vi "Begin.vi"   [LabVIEW 2020]
doc: "Called before other user functions, this VI is expected to open initial I/O refnums, load in file data, and do all program initialization. Notice that the <B>error out</B> terminal is simply used for data flow. Wiring it to other structures or subVIs ensures that this VI runs first."
uses:
  <vilib>/Rock Robotics/WPI/DriverStation/WPI_DriverStationRobotMode2.ctl
  <vilib>/Rock Robotics/WPI/Joystick/WPI_JoystickDeviceEnum.ctl
  <vilib>/Rock Robotics/WPI/ThirdParty/REV Robotics/REVLib/Typedef/Spark MAX Control Type.ctl
  Robot Global Data.vi
  <vilib>/Rock Robotics/WPI/ThirdParty/Phoenix-LabVIEW/CANCoder/Get/CTRE_Phoenix_CANcoder_GetSensorData.vi
  <vilib>/Rock Robotics/WPI/ThirdParty/Phoenix-LabVIEW/CANCoder/Set/CTRE_Phoenix_CANcoder_SetPosition.vi
types:
  T1 = typedef "Spark MAX Control Type.ctl" = enum16{"Percent VBus", "Voltage", "Velocity", "Position", "Smart Motion", "Current", "Smart Velocity"}
  T2 = typedef "WPI_JoystickDeviceEnum.ctl" = enum16{"USB 0", "USB 1", "USB 2", "USB 3", "USB 4", "USB 5"}
  T3 = typedef "WPI_DriverStationRobotMode2.ctl" = enum16{"Autonomous Disabled", "Autonomous Enabled", "Teleop Disabled", "Teleop Enabled", "Disconnected", "Finish", "Test Disabled", "Test Enabled", "Emergency Stopped"}
  T4 = typedef "WPI_MotorControlDeviceRef.ctl" = cluster{"DeviceStatus":errorcluster, "Type":T5, "PWM":cluster{"PWM Channel":T6, "DeadBand":T7}, "CAN":cluster{"Device Number":u8, "SetOutput VI Ref":variant, "GetOutput VI Ref":variant, "Enable VI Ref":variant, "Disable VI Ref":variant, "Data":variant}, "Invert":bool, "DIO PWM":cluster{"PWM \"Enable\" Channel":T6, "DIOChannel":T8, "PWM Rate":dbl}}
  T5 = typedef "WPI_MotorControlType.ctl" = enum16{"PWM", "CAN", "DIO PWM"}
  T6 = typedef "FPGA_DIOPWMChannel.ctl" = enum8{"PWM 0", "PWM 1", "PWM 2", "PWM 3", "PWM 4", "PWM 5", "PWM 6", "PWM 7", "PWM 8", "PWM 9", "PWM MXP 0", "PWM MXP 1", "PWM MXP 2", "PWM MXP 3", "PWM MXP 4", "PWM MXP 5", "PWM MXP 6", "PWM MXP 7", "PWM MXP 8", "PWM MXP 9", "Invalid"}
  T7 = typedef "WPI_PWMDeadband.ctl" = cluster{"Name":string, "maxPositivePwm":i32, "minPositivePwm":i32, "centerPwm":i32, "maxNegativePwm":i32, "minNegativePwm":i32, "angularRange":u16}
  T8 = typedef "FPGA_DIOChannel.ctl" = enum8{"DIO 0", "DIO 1", "DIO 2", "DIO 3", "DIO 4", "DIO 5", "DIO 6", "DIO 7", "DIO 8", "DIO 9", "DIO MXP 0", "DIO MXP 1", "DIO MXP 2", "DIO MXP 3", "DIO MXP 4", "DIO MXP 5", "DIO MXP 6", "DIO MXP 7", "DIO MXP 8", "DIO MXP 9", "DIO MXP 10", "DIO MXP 11", "DIO MXP 12", "DIO MXP 13", "DIO MXP 14", "DIO MXP 15", "SPI Port CS1", "SPI Port CS2", "SPI Port CS3", "SPI Port MISO", "SPI Port MOSI", "Invalid"}
  T9 = typedef "CTRE_Phoenix_CANcoder_DeviceRef.ctl" = cluster{"DeviceStatus":errorcluster, "Device Number":u8, "Handle":u64, "UsageFrame":u32, "Library Path":path}
  T10 = typedef "WPI_JoystickDevRef.ctl" = cluster{"Device":T2}
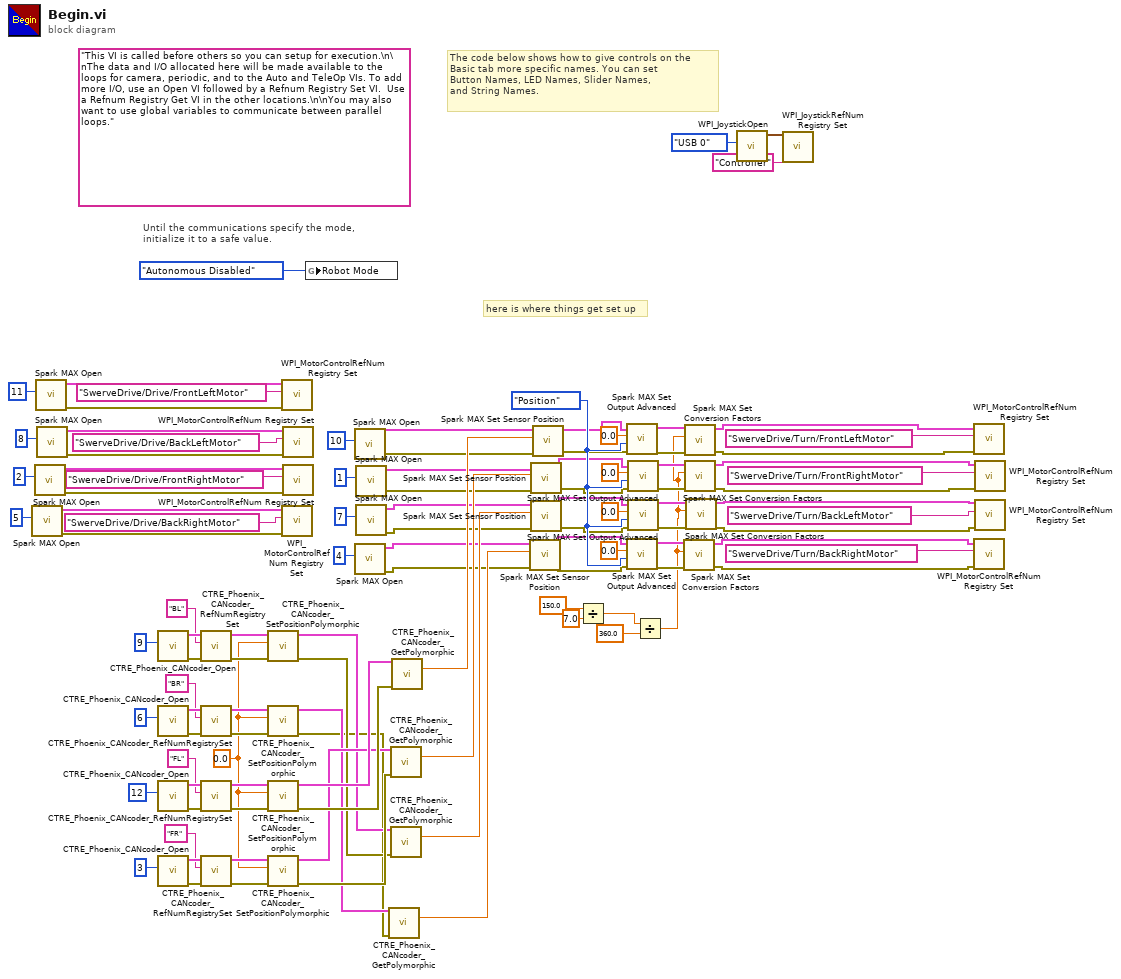
[diagram p0: block diagram]
diagram:
  w1 = 0.0 ("Setpoint")
  w63 = Spark_MAX_Control_Type."Position" ("Control Mode")
  (unwired) "This VI is called before others so you can setup for execution.\n\nThe data and I/O allocated here will be made available to the loops for camera, periodic, and to the Auto and TeleOp VIs. To add more I/O, use an Open VI followed by a Refnum Registry Set VI.  Use a Refnum Registry Get VI in the other locations.\n\nYou may also want to use global variables to communicate between parallel loops."
  # "here is where things get set up"
  # "The code below shows how to give controls on the\nBasic tab more specific names. You can set\nButton Names, LED Names, Slider Names,\nand String Names."
  # "Until the communications specify the mode,\ninitialize it to a safe value."
  n1 = call <vilib>:"Spark MAX Open.vi"("Device Number"=u8 5) -> ("error out"=w93:errorcluster, "MotorControlDeviceRef"=w92:T4)  [unwired: 9 in]
  n2 = call <vilib>:"Spark MAX Open.vi"("Device Number"=u8 2) -> ("error out"=w96:errorcluster, "MotorControlDeviceRef"=w95:T4)  [unwired: 9 in]
  n3 = call <vilib>:"Spark MAX Open.vi"("Device Number"=u8 11) -> ("error out"=w102:errorcluster, "MotorControlDeviceRef"=w101:T4)  [unwired: 9 in]
  n4 = call <vilib>:"Spark MAX Open.vi"("Device Number"=u8 8) -> ("error out"=w99:errorcluster, "MotorControlDeviceRef"=w98:T4)  [unwired: 9 in]
  n5 = call <vilib>:"CTRE_Phoenix_CANcoder_Open.vi"("Device Number"=u8 9) -> ("error out"=w78:errorcluster, "CTRE_CANcoder_DeviceRef"=w77:T9)  [unwired: 9 in]
  n6 = call <vilib>:"CTRE_Phoenix_CANcoder_Open.vi"("Device Number"=u8 6) -> ("error out"=w74:errorcluster, "CTRE_CANcoder_DeviceRef"=w73:T9)  [unwired: 9 in]
  n7 = call <vilib>:"CTRE_Phoenix_CANcoder_Open.vi"("Device Number"=u8 12) -> ("error out"=w86:errorcluster, "CTRE_CANcoder_DeviceRef"=w85:T9)  [unwired: 9 in]
  n8 = call <vilib>:"CTRE_Phoenix_CANcoder_Open.vi"("Device Number"=u8 3) -> ("error out"=w82:errorcluster, "CTRE_CANcoder_DeviceRef"=w81:T9)  [unwired: 9 in]
  n9 = call <vilib>:"CTRE_Phoenix_CANcoder_RefNumRegistrySet.vi"("error in (no error)"=w78, "refnum name"="BL", "CTRE_CANcoder_DeviceRef"=w77) -> ("error out"=w5:errorcluster, "CTRE_CANcoder_DeviceRef"=w4:T9)  [unwired: 7 in]
  n10 = call <vilib>:"CTRE_Phoenix_CANcoder_RefNumRegistrySet.vi"("error in (no error)"=w74, "refnum name"="BR", "CTRE_CANcoder_DeviceRef"=w73) -> ("error out"=w7:errorcluster, "CTRE_CANcoder_DeviceRef"=w6:T9)  [unwired: 7 in]
  n11 = call <vilib>:"CTRE_Phoenix_CANcoder_RefNumRegistrySet.vi"("error in (no error)"=w86, "refnum name"="FL", "CTRE_CANcoder_DeviceRef"=w85) -> ("error out"=w16:errorcluster, "CTRE_CANcoder_DeviceRef"=w17:T9)  [unwired: 7 in]
  n12 = call <vilib>:"CTRE_Phoenix_CANcoder_RefNumRegistrySet.vi"("error in (no error)"=w82, "refnum name"="FR", "CTRE_CANcoder_DeviceRef"=w81) -> ("error out"=w3:errorcluster, "CTRE_CANcoder_DeviceRef"=w2:T9)  [unwired: 7 in]
  n13 = call-poly <vilib>:"CTRE_Phoenix_CANcoder_SetPositionPolymorphic.vi"("error in (no error)"=w5, "Position"=w1, "CTRE_CANcoder_DeviceRef"=w4) -> ("error out"=w10:errorcluster, "CTRE_CANcoder_DeviceRef"=w11:T9)  [unwired: 7 in]
  n14 = call-poly <vilib>:"CTRE_Phoenix_CANcoder_SetPositionPolymorphic.vi"("error in (no error)"=w7, "Position"=w1, "CTRE_CANcoder_DeviceRef"=w6) -> ("error out"=w8:errorcluster, "CTRE_CANcoder_DeviceRef"=w9:T9)  [unwired: 7 in]
  n15 = call-poly <vilib>:"CTRE_Phoenix_CANcoder_SetPositionPolymorphic.vi"("error in (no error)"=w16, "Position"=w1, "CTRE_CANcoder_DeviceRef"=w17) -> ("error out"=w15:errorcluster, "CTRE_CANcoder_DeviceRef"=w14:T9)  [unwired: 7 in]
  n16 = call-poly <vilib>:"CTRE_Phoenix_CANcoder_SetPositionPolymorphic.vi"("error in (no error)"=w3, "Position"=w1, "CTRE_CANcoder_DeviceRef"=w2) -> ("error out"=w12:errorcluster, "CTRE_CANcoder_DeviceRef"=w13:T9)  [unwired: 7 in]
  n17 = call <vilib>:"WPI_MotorControlRefNum Registry Set.vi"("error in (no error)"=w102, "refnum name"="SwerveDrive/Drive/FrontLeftMotor", "MotorControlDevRef"=w101) -> ()  [unwired: 7 in, 2 out]
  n18 = call <vilib>:"WPI_MotorControlRefNum Registry Set.vi"("error in (no error)"=w93, "refnum name"="SwerveDrive/Drive/BackRightMotor", "MotorControlDevRef"=w92) -> ()  [unwired: 7 in, 2 out]
  n19 = call <vilib>:"WPI_MotorControlRefNum Registry Set.vi"("error in (no error)"=w99, "refnum name"="SwerveDrive/Drive/BackLeftMotor", "MotorControlDevRef"=w98) -> ()  [unwired: 7 in, 2 out]
  n20 = call <vilib>:"WPI_MotorControlRefNum Registry Set.vi"("error in (no error)"=w96, "refnum name"="SwerveDrive/Drive/FrontRightMotor", "MotorControlDevRef"=w95) -> ()  [unwired: 7 in, 2 out]
  n21 = global write "Robot Global Data.vi" "Robot Mode"(WPI_DriverStationRobotMode2."Autonomous Disabled" ("Robot Mode")) -> ()
  n22 = call <vilib>:"Spark MAX Open.vi"("Device Number"=u8 10) -> ("error out"=w24:errorcluster, "MotorControlDeviceRef"=w25:T4)  [unwired: 9 in]
  n23 = call <vilib>:"Spark MAX Open.vi"("Device Number"=u8 4) -> ("error out"=w18:errorcluster, "MotorControlDeviceRef"=w19:T4)  [unwired: 9 in]
  n24 = call <vilib>:"Spark MAX Open.vi"("Device Number"=u8 1) -> ("error out"=w22:errorcluster, "MotorControlDeviceRef"=w23:T4)  [unwired: 9 in]
  n25 = call <vilib>:"Spark MAX Open.vi"("Device Number"=u8 7) -> ("error out"=w20:errorcluster, "MotorControlDeviceRef"=w21:T4)  [unwired: 9 in]
  n26 = call-poly <vilib>:"CTRE_Phoenix_CANcoder_GetPolymorphic.vi"("CTRE_CANcoder_DeviceRef"=w9, "error in"=w8) -> ("Position"=w47:dbl)  [unwired: 9 in, 4 out]
  n27 = call-poly <vilib>:"CTRE_Phoenix_CANcoder_GetPolymorphic.vi"("CTRE_CANcoder_DeviceRef"=w13, "error in"=w12) -> ("Position"=w49:dbl)  [unwired: 9 in, 4 out]
  n28 = call-poly <vilib>:"CTRE_Phoenix_CANcoder_GetPolymorphic.vi"("CTRE_CANcoder_DeviceRef"=w11, "error in"=w10) -> ("Position"=w48:dbl)  [unwired: 9 in, 4 out]
  n29 = call-poly <vilib>:"CTRE_Phoenix_CANcoder_GetPolymorphic.vi"("CTRE_CANcoder_DeviceRef"=w14, "error in"=w15) -> ("Position"=w50:dbl)  [unwired: 9 in, 4 out]
  n30 = call <vilib>:"Spark MAX Set Sensor Position.vi"("error in"=w18, "Position"=w47, "MotorControlDeviceRef"=w19) -> ("error out"=w51:errorcluster, "MotorControlDeviceRef"=w52:T4)  [unwired: 7 in]
  n31 = call <vilib>:"Spark MAX Set Sensor Position.vi"("error in"=w22, "Position"=w49, "MotorControlDeviceRef"=w23) -> ("error out"=w55:errorcluster, "MotorControlDeviceRef"=w56:T4)  [unwired: 7 in]
  n32 = call <vilib>:"Spark MAX Set Sensor Position.vi"("error in"=w20, "Position"=w48, "MotorControlDeviceRef"=w21) -> ("error out"=w53:errorcluster, "MotorControlDeviceRef"=w54:T4)  [unwired: 7 in]
  n33 = call <vilib>:"Spark MAX Set Sensor Position.vi"("error in"=w24, "Position"=w50, "MotorControlDeviceRef"=w25) -> ("error out"=w57:errorcluster, "MotorControlDeviceRef"=w58:T4)  [unwired: 7 in]
  n34 = Divide(x=150.0, y=7.0) -> (x/y=w27:dbl)
  n35 = call <vilib>:"Spark MAX Set Output Advanced.vi"("error in (no error)"=w57, "Control Mode"=w63, "Setpoint"=0.0, "MotorControlDevRef"=w58) -> ("error out"=w45:errorcluster, "MotorControlDevRef"=w46:T4)  [unwired: 6 in]
  n36 = call <vilib>:"Spark MAX Set Output Advanced.vi"("error in (no error)"=w51, "Control Mode"=w63, "Setpoint"=0.0, "MotorControlDevRef"=w52) -> ("error out"=w39:errorcluster, "MotorControlDevRef"=w40:T4)  [unwired: 6 in]
  n37 = call <vilib>:"Spark MAX Set Output Advanced.vi"("error in (no error)"=w55, "Control Mode"=w63, "Setpoint"=0.0, "MotorControlDevRef"=w56) -> ("error out"=w43:errorcluster, "MotorControlDevRef"=w44:T4)  [unwired: 6 in]
  n38 = call <vilib>:"Spark MAX Set Output Advanced.vi"("error in (no error)"=w53, "Control Mode"=w63, "Setpoint"=0.0, "MotorControlDevRef"=w54) -> ("error out"=w41:errorcluster, "MotorControlDevRef"=w42:T4)  [unwired: 6 in]
  n39 = Divide(x=w27, y=360.0) -> (x/y=w26:dbl)
  n40 = call <vilib>:"Spark MAX Set Conversion Factors.vi"("error in (no error)"=w39, "Position Factor (1)"=w26, "MotorControlDeviceRef in"=w40) -> ("error out"=w31:errorcluster, "MotorControlDeviceRef out"=w32:T4)  [unwired: 7 in]
  n41 = call <vilib>:"Spark MAX Set Conversion Factors.vi"("error in (no error)"=w45, "Position Factor (1)"=w26, "MotorControlDeviceRef in"=w46) -> ("error out"=w37:errorcluster, "MotorControlDeviceRef out"=w38:T4)  [unwired: 7 in]
  n42 = call <vilib>:"Spark MAX Set Conversion Factors.vi"("error in (no error)"=w43, "Position Factor (1)"=w26, "MotorControlDeviceRef in"=w44) -> ("error out"=w35:errorcluster, "MotorControlDeviceRef out"=w36:T4)  [unwired: 7 in]
  n43 = call <vilib>:"Spark MAX Set Conversion Factors.vi"("error in (no error)"=w41, "Position Factor (1)"=w26, "MotorControlDeviceRef in"=w42) -> ("error out"=w33:errorcluster, "MotorControlDeviceRef out"=w34:T4)  [unwired: 7 in]
  n44 = call <vilib>:"WPI_JoystickOpen.vi"("JoystickDevice"=WPI_JoystickDeviceEnum."USB 0") -> ("JoystickDevRef"=w105:T10)  [unwired: 10 in]
  n45 = call <vilib>:"WPI_JoystickRefNum Registry Set.vi"("refnum name"="Controller", "JoystickDevRef"=w105) -> ()  [unwired: 8 in, 2 out]
  n46 = call <vilib>:"WPI_MotorControlRefNum Registry Set.vi"("error in (no error)"=w37, "refnum name"="SwerveDrive/Turn/FrontLeftMotor", "MotorControlDevRef"=w38) -> ()  [unwired: 7 in, 2 out]
  n47 = call <vilib>:"WPI_MotorControlRefNum Registry Set.vi"("error in (no error)"=w31, "refnum name"="SwerveDrive/Turn/BackRightMotor", "MotorControlDevRef"=w32) -> ()  [unwired: 7 in, 2 out]
  n48 = call <vilib>:"WPI_MotorControlRefNum Registry Set.vi"("error in (no error)"=w35, "refnum name"="SwerveDrive/Turn/FrontRightMotor", "MotorControlDevRef"=w36) -> ()  [unwired: 7 in, 2 out]
  n49 = call <vilib>:"WPI_MotorControlRefNum Registry Set.vi"("error in (no error)"=w33, "refnum name"="SwerveDrive/Turn/BackLeftMotor", "MotorControlDevRef"=w34) -> ()  [unwired: 7 in, 2 out]
